vi "探头温度显示.vi"(11 "校准参数":u16(ring) caption="校准参数：" items=["pH", "DO", "浊度", "电导率", "叶绿素a", "藻密度", "ORP", "DO2", "氯化物"]) -> (3 "温度数据":sgl, 5 "温度偏移修正值":sgl)   [LabVIEW 2022 SP3, in "斯坦道多参数.lvlib"]
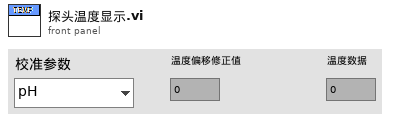
[diagram p1: front panel]
types:
  T1 = typedef "斯坦道多参数.lvlib/探头类型.ctl" = enum16{"禹山", "国弘", "纳清", "STD"}
  T2 = cluster{"pH探头选择":T1, "DO探头选择":T1, "电导率探头选择":T1, "浊度探头选择":T1, "悬浮物探头选择":T1, "叶绿素a探头选择":T1, "蓝绿藻探头选择":T1, "orp探头选择":T1, "COD探头选择":T1, "DO2探头选择":T1, "氨氮探头选择":T1, "水中油探头选择":T1, "余氯探头选择":T1}
  T3 = cluster{"电极状态标志":u16, "电极型号标志":u16, "酸碱度测量值":sgl, "温度测量值":sgl, "酸碱度信号值":sgl, "温度信号值":sgl, "酸碱度偏移修正值":sgl, "温度偏移修正值":sgl, "手动温度补偿值":sgl, "酸碱度电极零点":sgl, "酸碱度电极斜率":sgl, "第1点标准值记录":sgl, "第1点信号值记录":sgl, "第1点温度值记录":sgl, "第2点标准值记录":sgl, "第2点信号值记录":sgl, "第2点温度值记录":sgl, "命令滤波设定":u16, "温度模式":enum16{"ATC", "MTC"}, "生产批次":u16, "电极序号":u16, "串口地址":u16, "串口波特率":enum16{"9600", "19200", "115200"}, "串口校验位":enum16{"NONE", "ODD", "EVEN"}, "串口停止位":enum16{"1bit", "2bit"}, "第一点标准值":sgl, "第二点标准值":sgl}
  T4 = cluster{"报警码":u16, "pH数值":sgl, "0X0003_NC":sgl, "温度数据":sgl, "pH原始信号 mv":sgl, "0X0009_NC":string, "产品名称":string, "序列号":string, "硬件版本":string, "软件版本":string, "通讯地址":u16, "波特率":u16, "设备类型":u16, "0X0026_NC":string, "第一点原始数据":sgl, "第一点校准数据":sgl, "第二点原始数据":sgl, "第二点校准数据":sgl, "探头校准命令":u16, "温度校准参数":sgl, "温度校准命令":u16}
  T5 = cluster{"电极状态标志":u16, "电极型号标志":u16, "溶解氧测量值":sgl, "温度测量值":sgl, "溶解氧饱和度值":sgl, "盐度补偿值":sgl, "大气压补偿值":sgl, "溶解氧偏移修正值":sgl, "温度偏移修正值":sgl, "手动温度补偿值":sgl, "溶解氧电极零点":sgl, "溶解氧电极斜率":sgl, "第1点标准值记录":sgl, "第1点信号值记录":sgl, "第1点温度值记录":sgl, "第2点标准值记录":sgl, "第2点信号值记录":sgl, "第2点温度值记录":sgl, "命令滤波设定":u16, "温度模式":enum16{"ATC", "MTC"}, "生产批次":u16, "电极序号":u16, "串口地址":u16, "串口波特率":enum16{"9600", "19200", "115200"}, "串口校验位":enum16{"NONE", "ODD", "EVEN"}, "串口停止位":enum16{"1bit", "2bit"}, "第一点标准值":sgl, "第二点标准值":sgl}
  T6 = cluster{"报警码":u16, "溶解氧数值（mg/L）":sgl, "溶解氧数据（%）":sgl, "温度数据":sgl, "溶解氧原始信号 nA":sgl, "大气压力":sgl, "盐度":sgl, "0X0009_NC":string, "产品名称":string, "序列号":string, "硬件版本":string, "软件版本":string, "通讯地址":u16, "波特率":u16, "设备类型":u16, "0X0026_NC":string, "第一点原始数据":sgl, "第一点校准数据":sgl, "第二点原始数据":sgl, "第二点校准数据":sgl, "探头校准命令":u16, "温度校准参数":sgl, "温度校准命令":u16}
  T7 = cluster{"电极状态标志":u16, "电极型号标志":u16, "浊度测量值":sgl, "温度测量值":sgl, "浊度信号值":sgl, "浊度偏移修正值":sgl, "温度偏移修正值":sgl, "手动温度补偿值":sgl, "浊度电极零点":sgl, "浊度电极斜率":sgl, "清洁周期":u16, "命令滤波设定":u16, "温度模式":enum16{"ATC", "MTC"}, "生产批次":u16, "电极序号":u16, "串口地址":u16, "串口波特率":enum16{"9600", "19200", "115200"}, "串口校验位":enum16{"NONE", "ODD", "EVEN"}, "串口停止位":enum16{"1bit", "2bit"}, "第一点标准值":sgl, "第二点标准值":sgl, "第三点标准值":sgl}
  T8 = cluster{"报警码":u16, "浊度数值 NTU":sgl, "温度数据":sgl, "原始光强数值":u16, "量程":u16, "平均次数":u16, "清扫模式":u16, "清扫次数":u16, "清扫间隔分钟":u16, "0X000B_NC":string, "产品名称":string, "序列号":string, "硬件版本":string, "软件版本":string, "通讯地址":u16, "波特率":u16, "设备类型":u16, "0X0026_NC":string, "校准量程":u16, "第一点原始光强":u16, "第一点校准数据":sgl, "第二点原始光强":u16, "第二点校准数据":sgl, "第三点原始光强":u16, "第三点校准数据":sgl, "探头校准命令":u16, "温度校准参数":sgl, "温度校准命令":u16}
  T9 = cluster{"电极状态标志":u16, "电极型号标志":u16, "电导率测量值":sgl, "温度测量值":sgl, "电导率信号值":sgl, "温度信号值":sgl, "温度补偿系数":sgl, "电导率偏移修正值":sgl, "温度偏移修正值":sgl, "手动温度补偿值":sgl, "电导率电极零点":sgl, "电导率电极斜率":sgl, "命令滤波设定":u16, "温度模式":enum16{"ATC", "MTC"}, "生产批次":u16, "电极序号":u16, "串口地址":u16, "串口波特率":enum16{"9600", "19200", "115200"}, "串口校验位":enum16{"NONE", "ODD", "EVEN"}, "串口停止位":enum16{"1bit", "2bit"}, "第一点标准值":sgl, "第二点标准值":sgl}
  T10 = cluster{"报警码":u16, "电导率数据（uS/cm）":sgl, "0x0003 NC":sgl, "温度数据":sgl, "电导率原始信号电阻":sgl, "当前量程":u16, "温度补偿系数":sgl, "0X0009_NC":string, "产品名称":string, "序列号":string, "硬件版本":string, "软件版本":string, "通讯地址":u16, "波特率":u16, "设备类型":u16, "0X0026_NC":string, "第一点原始数据":sgl, "第一点校准数据":sgl, "0X0035_NC":sgl, "0X0037_NC":sgl, "探头校准命令":u16, "温度校准参数":sgl, "温度校准命令":u16}
  T11 = cluster{"报警码":u16, "叶绿素a":sgl, "温度数据":sgl, "原始光强数值":u16, "量程":u16, "平均次数":u16, "清扫模式":u16, "清扫次数":u16, "清扫间隔分钟":u16, "0X000B_NC":string, "产品名称":string, "序列号":string, "硬件版本":string, "软件版本":string, "通讯地址":u16, "波特率":u16, "设备类型":u16, "0X0026_NC":string, "校准量程":u16, "第一点原始光强":u16, "第一点校准数据":sgl, "第二点原始光强":u16, "第二点校准数据":sgl, "第三点原始光强":u16, "第三点校准数据":sgl, "探头校准命令":u16, "温度校准参数":sgl, "温度校准命令":u16}
  T12 = cluster{"报警码":u16, "蓝绿藻":sgl, "温度数据":sgl, "原始光强数值":u16, "量程":u16, "平均次数":u16, "清扫模式":u16, "清扫次数":u16, "清扫间隔分钟":u16, "0X000B_NC":string, "产品名称":string, "序列号":string, "硬件版本":string, "软件版本":string, "通讯地址":u16, "波特率":u16, "设备类型":u16, "0X0026_NC":string, "校准量程":u16, "第一点原始光强":u16, "第一点校准数据":sgl, "第二点原始光强":u16, "第二点校准数据":sgl, "第三点原始光强":u16, "第三点校准数据":sgl, "探头校准命令":u16, "温度校准参数":sgl, "温度校准命令":u16}
  T13 = cluster{"电极状态标志":u16, "电极型号标志":u16, "测量值":sgl, "温度测量值":sgl, "信号值":sgl, "温度信号值":sgl, "000AH_NC":sgl, "偏移修正值":sgl, "温度偏移修正值":sgl, "手动温度补偿值":sgl, "命令滤波设定":u16, "温度模式":enum16{"ATC", "MTC"}, "生产批次":u16, "传感器序号":u16, "串口地址":u16, "串口波特率":enum16{"9600", "19200", "115200"}, "串口校验位":enum16{"NONE", "ODD", "EVEN"}, "串口停止位":enum16{"1bit", "2bit"}}
  T14 = cluster{"电极状态标志":u16, "电极型号标志":u16, "测量值":sgl, "温度测量值":sgl, "信号值":sgl, "温度信号值":sgl, "偏移修正值":sgl, "温度偏移修正值":sgl, "手动温度补偿值":sgl, "电极零点":sgl, "电极斜率":sgl, "第1点标准值记录":sgl, "第1点信号值记录":sgl, "第1点温度值记录":sgl, "第2点标准值记录":sgl, "第2点信号值记录":sgl, "第2点温度值记录":sgl, "命令滤波设定":u16, "温度模式":enum16{"ATC", "MTC"}, "生产批次":u16, "电极序号":u16, "串口地址":u16, "串口波特率":enum16{"9600", "19200", "115200"}, "串口校验位":enum16{"NONE", "ODD", "EVEN"}, "串口停止位":enum16{"1bit", "2bit"}, "第一点标准值":sgl, "第二点标准值":sgl}
  T15 = cluster{"报警码":u16, "参数1数据":sgl, "参数2数据":sgl, "参数3数据":sgl, "参数4数据":sgl, "温度数据":sgl, "参数1原始信号":sgl, "参数2原始信号":sgl, "参数3原始信号":sgl, "参数4原始信号":sgl, "序列号":string, "硬件版本":string, "软件版本":string, "通讯地址":u16, "波特率":u16, "设备类型":u16, "0X0026_NC":string, "校准参数类型":u16, "第一点原始数据":sgl, "第一点校准数据":sgl, "第二点原始数据":sgl, "第二点校准数据":sgl, "探头校准命令":u16, "温度校准参数":sgl, "温度校准命令":u16}
  T16 = cluster{"电极状态标志":u16, "电极型号标志":u16, "测量值":sgl, "温度测量值":sgl, "信号值":sgl, "水中油B值":sgl, "温度B值":sgl, "水中油零点系数":sgl, "水中油斜率系数":sgl, "水中油K值":sgl, "空白电位值":sgl, "温度信号值":sgl, "温度补偿系数":sgl, "测量档位":u16, "清洁周期":u16, "命令寄存器":u16, "数位滤波设定":u16, "温度模式":enum16{"ATC", "MTC"}, "生产批次":u16, "电极序号":u16, "串口地址":u16, "串口波特率":enum16{"9600", "19200", "115200"}, "串口校验位":enum16{"NONE", "ODD", "EVEN"}, "串口停止位":enum16{"1bit", "2bit"}, "第一点校正指令":u16, "第一点标准值":sgl, "第二点校正指令":u16, "第二点标准值":sgl, "第三点校正指令":u16, "第三点标准值":sgl}
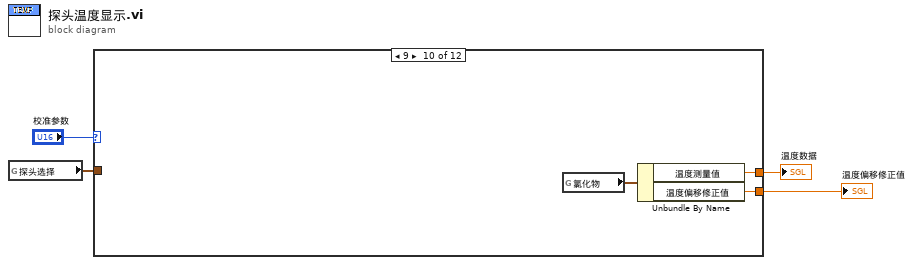
[diagram p0: block diagram]
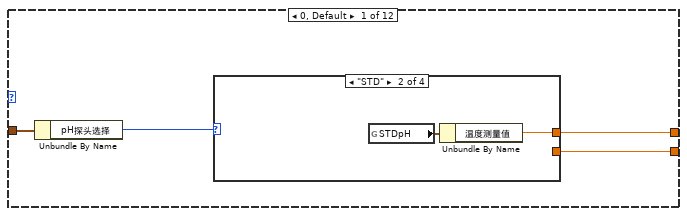
[diagram p2: hidden frame]
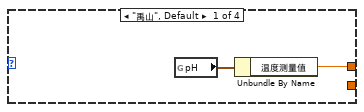
[diagram p3: hidden frame]
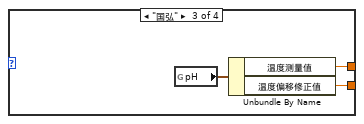
[diagram p4: hidden frame]
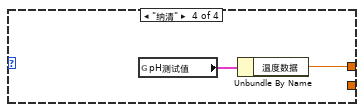
[diagram p5: hidden frame]
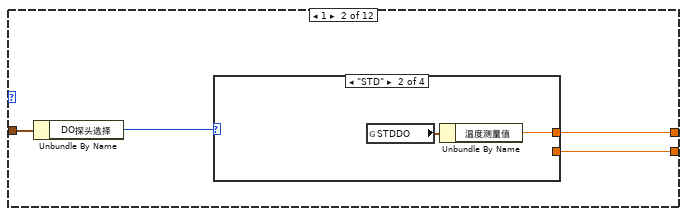
[diagram p6: hidden frame]
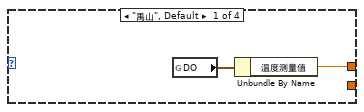
[diagram p7: hidden frame]
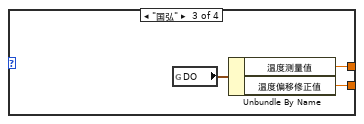
[diagram p8: hidden frame]
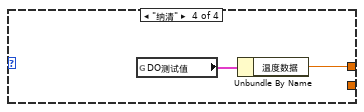
[diagram p9: hidden frame]
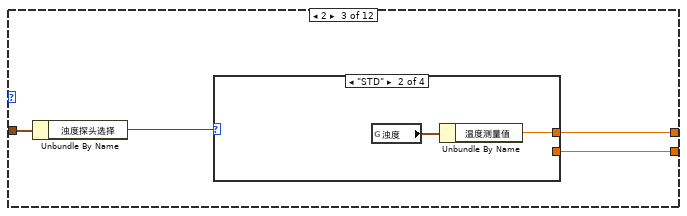
[diagram p10: hidden frame]
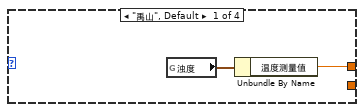
[diagram p11: hidden frame]
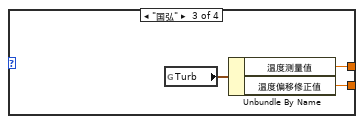
[diagram p12: hidden frame]
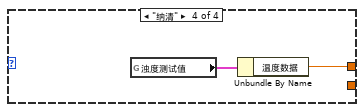
[diagram p13: hidden frame]
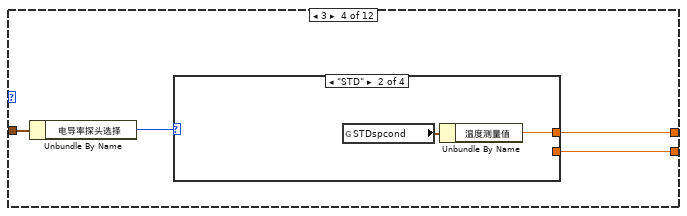
[diagram p14: hidden frame]
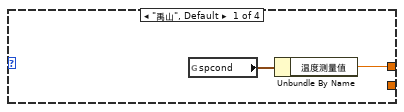
[diagram p15: hidden frame]
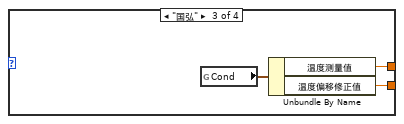
[diagram p16: hidden frame]
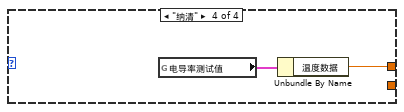
[diagram p17: hidden frame]
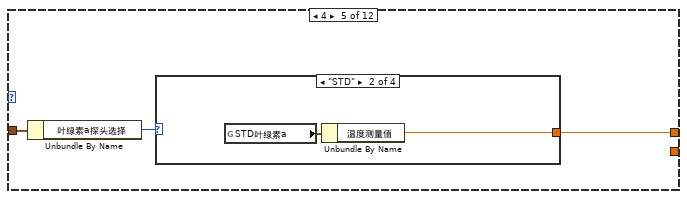
[diagram p18: hidden frame]
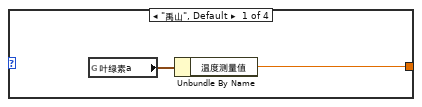
[diagram p19: hidden frame]
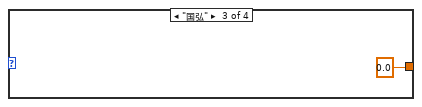
[diagram p20: hidden frame]
diagram:
  n1 = global read "断电保存变量.vi" "探头选择"() -> (w2:T2)
  n2 = case shown="9" "校准参数" {
    tunnel: [w7 w20 w33 w46 w58 w68 w78 w86 w88 w91 w93 w96] -> w4
    tunnel: w2 -> [w6 w19 w32 w45 w57 w67 w77 _ _ _ _ _]
    tunnel: [w5 w18 w31 w44 _ _ w76 _ _ w90 _ w95] -> w1
    frame 0, Default {
      n3 = Unbundle By Name(w6) -> ("pH探头选择"=w8:T1)
      n4 = case shown="\"STD\"" w8 {
        tunnel: [w9 w11 w14 w17] -> w7
        tunnel: [_ _ w13 _] -> w5
        frame "禹山", Default {
          n5 = global read "禹山过程全局变量.vi" "pH"() -> (w10:cluster{"温度测量值":sgl, "ORP":sgl, "pH":sgl})
          n6 = Unbundle By Name(w10) -> ("温度测量值"=w9:sgl)
        }
        frame "STD" {
          n7 = global read "禹山过程全局变量.vi" "STDpH"() -> (w12:cluster{"温度测量值":sgl, "pH":sgl, "信号值":sgl})
          n8 = Unbundle By Name(w12) -> ("温度测量值"=w11:sgl)
        }
        frame "国弘" {
          n9 = global read "国弘过程全局变量.vi" "pH"() -> (w15:T3)
          n10 = Unbundle By Name(w15) -> ("温度测量值"=w14:sgl, "温度偏移修正值"=w13:sgl)
        }
        frame "纳清" {
          n11 = global read "纳清过程全局变量.vi" "pH测试值"() -> (w16:T4)
          n12 = Unbundle By Name(w16) -> ("温度数据"=w17:sgl)
        }
      }
    }
    frame 1 {
      n13 = Unbundle By Name(w19) -> ("DO探头选择"=w21:T1)
      n14 = case shown="\"STD\"" w21 {
        tunnel: [w22 w24 w27 w30] -> w20
        tunnel: [_ _ w26 _] -> w18
        frame "禹山", Default {
          n15 = global read "禹山过程全局变量.vi" "DO"() -> (w23:cluster{"温度测量值":sgl, "DO%":sgl, "DOmg/L":sgl})
          n16 = Unbundle By Name(w23) -> ("温度测量值"=w22:sgl)
        }
        frame "STD" {
          n17 = global read "禹山过程全局变量.vi" "STDDO"() -> (w25:cluster{"温度测量值":sgl, "DO%":sgl, "DOmg/L":sgl})
          n18 = Unbundle By Name(w25) -> ("温度测量值"=w24:sgl)
        }
        frame "国弘" {
          n19 = global read "国弘过程全局变量.vi" "DO"() -> (w28:T5)
          n20 = Unbundle By Name(w28) -> ("温度测量值"=w27:sgl, "温度偏移修正值"=w26:sgl)
        }
        frame "纳清" {
          n21 = global read "纳清过程全局变量.vi" "DO测试值"() -> (w29:T6)
          n22 = Unbundle By Name(w29) -> ("温度数据"=w30:sgl)
        }
      }
    }
    frame 2 {
      n23 = Unbundle By Name(w32) -> ("浊度探头选择"=w34:T1)
      n24 = case shown="\"STD\"" w34 {
        tunnel: [w35 w37 w40 w43] -> w33
        tunnel: [_ _ w39 _] -> w31
        frame "禹山", Default {
          n25 = global read "禹山过程全局变量.vi" "浊度"() -> (w36:cluster{"温度测量值":sgl, "浊度测量值":sgl})
          n26 = Unbundle By Name(w36) -> ("温度测量值"=w35:sgl)
        }
        frame "STD" {
          n27 = global read "禹山过程全局变量.vi" "浊度"() -> (w38:cluster{"温度测量值":sgl, "浊度测量值":sgl})
          n28 = Unbundle By Name(w38) -> ("温度测量值"=w37:sgl)
        }
        frame "国弘" {
          n29 = global read "国弘过程全局变量.vi" "Turb"() -> (w41:T7)
          n30 = Unbundle By Name(w41) -> ("温度测量值"=w40:sgl, "温度偏移修正值"=w39:sgl)
        }
        frame "纳清" {
          n31 = global read "纳清过程全局变量.vi" "浊度测试值"() -> (w42:T8)
          n32 = Unbundle By Name(w42) -> ("温度数据"=w43:sgl)
        }
      }
    }
    frame 3 {
      n33 = Unbundle By Name(w45) -> ("电导率探头选择"=w47:T1)
      n34 = case shown="\"STD\"" w47 {
        tunnel: [w48 w50 w53 w56] -> w46
        tunnel: [_ _ w52 _] -> w44
        frame "禹山", Default {
          n35 = global read "禹山过程全局变量.vi" "spcond"() -> (w49:cluster{"温度测量值":sgl, "测量值":sgl, "错误标志":u16})
          n36 = Unbundle By Name(w49) -> ("温度测量值"=w48:sgl)
        }
        frame "STD" {
          n37 = global read "禹山过程全局变量.vi" "STDspcond"() -> (w51:cluster{"温度测量值":sgl, "测量值":sgl, "信号值":sgl})
          n38 = Unbundle By Name(w51) -> ("温度测量值"=w50:sgl)
        }
        frame "国弘" {
          n39 = global read "国弘过程全局变量.vi" "Cond"() -> (w54:T9)
          n40 = Unbundle By Name(w54) -> ("温度测量值"=w53:sgl, "温度偏移修正值"=w52:sgl)
        }
        frame "纳清" {
          n41 = global read "纳清过程全局变量.vi" "电导率测试值"() -> (w55:T10)
          n42 = Unbundle By Name(w55) -> ("温度数据"=w56:sgl)
        }
      }
    }
    frame 4 {
      n43 = Unbundle By Name(w57) -> ("叶绿素a探头选择"=w59:T1)
      n44 = case shown="\"STD\"" w59 {
        tunnel: [w60 w62 sgl 0.0 ("温度数据") w66] -> w58
        frame "禹山", Default {
          n45 = global read "禹山过程全局变量.vi" "叶绿素a"() -> (w61:cluster{"温度测量值":sgl, "叶绿素测量值":sgl, "错误标志":u16})
          n46 = Unbundle By Name(w61) -> ("温度测量值"=w60:sgl)
        }
        frame "STD" {
          n47 = global read "禹山过程全局变量.vi" "STD叶绿素a"() -> (w63:cluster{"温度测量值":sgl, "叶绿素测量值":sgl, "信号值":sgl})
          n48 = Unbundle By Name(w63) -> ("温度测量值"=w62:sgl)
        }
        frame "国弘" {
        }
        frame "纳清" {
          n49 = global read "纳清过程全局变量.vi" "叶绿素a测试值"() -> (w65:T11)
          n50 = Unbundle By Name(w65) -> ("温度数据"=w66:sgl)
        }
      }
    }
    frame 5 {
      n51 = Unbundle By Name(w67) -> ("蓝绿藻探头选择"=w69:T1)
      n52 = case shown="\"国弘\"" w69 {
        tunnel: [sgl 0.0 ("温度数据") w71 sgl 0.0 ("温度数据") w75] -> w68
        frame "禹山", Default {
        }
        frame "STD" {
          n53 = global read "禹山过程全局变量.vi" "STD叶绿素a"() -> (w72:cluster{"温度测量值":sgl, "叶绿素测量值":sgl, "信号值":sgl})
          n54 = Unbundle By Name(w72) -> ("温度测量值"=w71:sgl)
        }
        frame "国弘" {
        }
        frame "纳清" {
          n55 = global read "纳清过程全局变量.vi" "蓝绿藻测试值"() -> (w74:T12)
          n56 = Unbundle By Name(w74) -> ("温度数据"=w75:sgl)
        }
      }
    }
    frame 6 {
      n57 = Unbundle By Name(w77) -> ("orp探头选择"=w79:T1)
      n58 = case shown="\"纳清\"" w79 {
        tunnel: [sgl 0.0 ("温度数据") w82 sgl 0.0 ("温度测量值")] -> w78
        tunnel: [_ w81 _] -> w76
        frame "禹山", Default {
        }
        frame "国弘" {
          n59 = global read "国弘过程全局变量.vi" "ORP"() -> (w83:T13)
          n60 = Unbundle By Name(w83) -> ("温度测量值"=w82:sgl, "温度偏移修正值"=w81:sgl)
        }
        frame "纳清" {
        }
      }
    }
    frame 7 {
      n61 = global read "禹山过程全局变量.vi" "DO 2"() -> (w85:cluster{"温度测量值":sgl, "DO%":sgl, "DOmg/L":sgl})
      n62 = Unbundle By Name(w85) -> ("温度测量值"=w86:sgl)
    }
    frame 8 {
      n63 = global read "禹山过程全局变量.vi" "DO 2"() -> (w87:cluster{"温度测量值":sgl, "DO%":sgl, "DOmg/L":sgl})
      n64 = Unbundle By Name(w87) -> ("温度测量值"=w88:sgl)
    }
    frame 9 {
      n65 = global read "国弘过程全局变量.vi" "氯化物"() -> (w89:T14)
      n66 = Unbundle By Name(w89) -> ("温度测量值"=w91:sgl, "温度偏移修正值"=w90:sgl)
    }
    frame 10 {
      n67 = global read "纳清过程全局变量.vi" "氨氮测试值"() -> (w92:T15)
      n68 = Unbundle By Name(w92) -> ("温度数据"=w93:sgl)
    }
    frame 11 {
      n69 = global read "国弘过程全局变量.vi" "水中油"() -> (w94:T16)
      n70 = Unbundle By Name(w94) -> ("温度测量值"=w96:sgl, "温度B值"=w95:sgl)
    }
  }
  "温度数据" <- w4
  "温度偏移修正值" <- w1
